vi "Status.vi"(7 "[x]":T1, 8 "error in (no error)":errorcluster, 11 "Serial Port in":refnum<visa-resource-name>) -> (0 "error out":errorcluster, 2 "Status":T2=enum."Pump Error", 3 "Serial Port out":refnum<visa-resource-name>)   [LabVIEW 2020, in "Chemyx_Syringe_Pump_driver.lvlib"]
doc: "Returns the current status of the pump. The status is returned as a status enum."
uses:
  Chemyx_Syringe_Pump_driver.lvlib
  controls/Pump_status_enum.ctl
  _private/Control/Control Mode.ctl
panel:
  # "Returns the current status of the pump. The status is returned as a status enum."
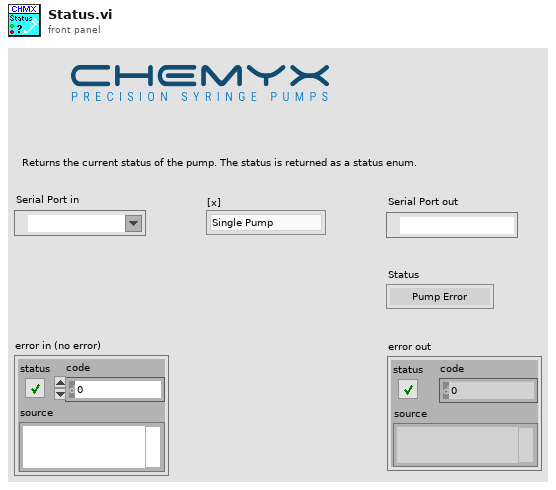
[diagram p1: front panel]
types:
  T1 = typedef "Chemyx_Syringe_Pump_driver.lvlib/Control Mode.ctl" = enum16{"Single Pump", "Pump Channel 1", "Pump Channel 2", "Cycle Mode"}
  T2 = typedef "Chemyx_Syringe_Pump_driver.lvlib/Pump_status_enum.ctl" = enum16{"Pump Idle", "Pump Running", "Pump Paused", "Pump Delay", "Pump Stalled", "Pump Error"}
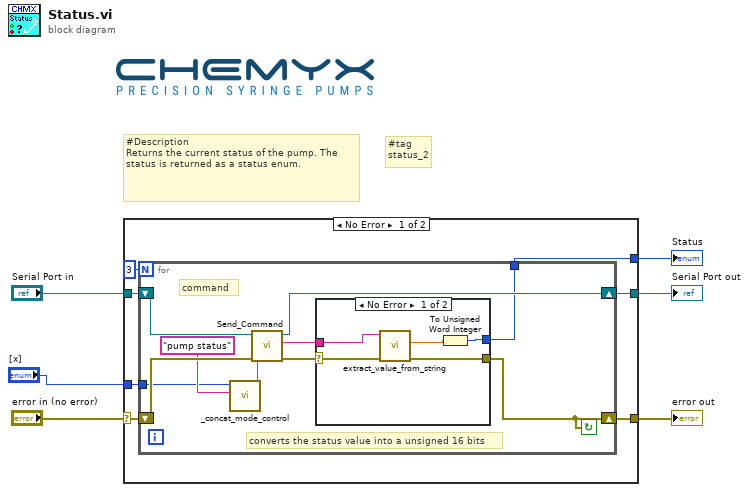
[diagram p0: block diagram]
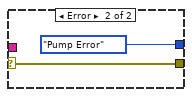
[diagram p2: hidden frame]
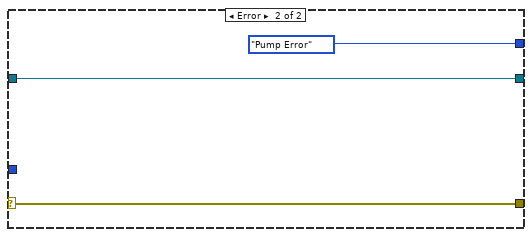
[diagram p3: hidden frame]
diagram:
  # "#tag\nstatus_2"
  # "#Description\nReturns the current status of the pump. The status is returned as a status enum."
  n1 = case shown="No Error" "error in (no error)" {
    selector: "error in (no error)" -> [w12 w33]
    tunnel: "Serial Port in" -> [w13 w32]
    tunnel: [w10 w33] -> w4
    tunnel: [w11 w32] -> w3
    tunnel: [w9 Pump_status_enum."Pump Error" ("Status")] -> w2
    tunnel: "[x]" -> [w8 _]
    frame No Error {
      n2 = for {
        N: 3 -> [_]
        tunnel: [w18] -> w9
        tunnel: w8 -> [w15]
        shift-right: [w21] -> w11
        shift-left: w13 -> [w23]
        shift-right: [w14] -> w10
        shift-left: w12 -> [w22]
        stop <- w14 continue-if-true
        # "converts the status value into a unsigned 16 bits"
        # "command"
        n3 = call "_concat_mode_control.vi"("write buffer"="pump status", "[x]"=w15) -> ("write buffer out"=w16:string)  [unwired: 9 in]
        n4 = call "Send_Command.vi"("error in (no error)"=w22, "write buffer"=w16, "Serial Port in"=w23) -> ("error out"=w20:errorcluster, "Read buffer"=w19:string, "VISA Refnum out"=w21:refnum<visa-resource-name>)  [unwired: 6 in]
        n5 = case shown="No Error" w20 {
          selector: w20 -> [w28 w30]
          tunnel: [w27 w30] -> w14
          tunnel: w19 -> [w26 _]
          tunnel: [w24 Pump_status_enum."Pump Error" ("Status")] -> w18
          frame No Error {
            n6 = call "extract_value_from_string.vi"("error in (no error)"=w28, "Input string"=w26) -> ("error out"=w27:errorcluster, "Value"=w25:dbl)  [unwired: 7 in, 1 out]
            n7 = To Unsigned Word Integer(number=w25) -> (unsigned 16bit integer=w24:u16)
          }
          frame Error {
          }
        }
      }
    }
    frame Error {
    }
  }
  "error out" <- w4
  "Serial Port out" <- w3
  "Status" <- w2
